vi "Deserialize Core.vi"(8 "error in (no error)":errorcluster, 10 "Serialized Attributes":string, 11 "Serialize in":refnum<class "Update Number Msg.lvclass">) -> (0 "error out":errorcluster, 3 "Serialize out":refnum<class "Update Number Msg.lvclass">)   [LabVIEW 2020, in "Chat Window.lvlib" / "Update Number Msg.lvclass"]
uses:
  Update Number Msg.lvclass
  Update Number Msg.lvclass/Update Number Msg.ctl
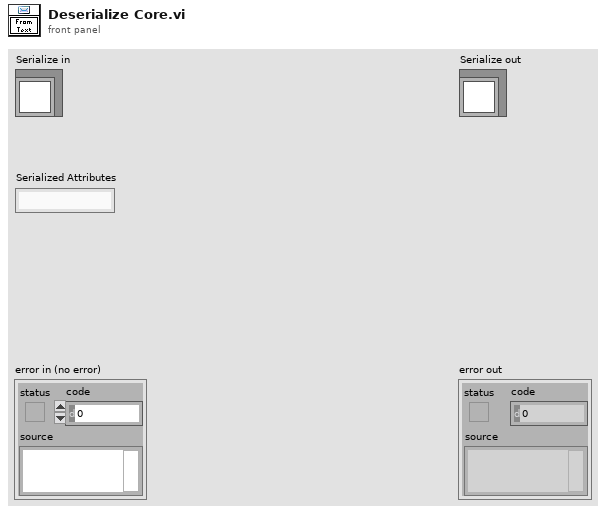
[diagram p1: front panel]
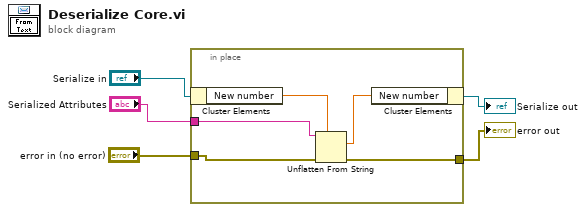
[diagram p0: block diagram]
diagram:
  n1 = in-place "In Place Element Structure" {
    in-place-border: "Serialized Attributes" -> [w9]
    in-place-border: "error in (no error)" -> [w8]
    in-place-border: [w6] -> w2
    n2 = in-place-cluster #1("Serialize in") -> ("New number"=w10:dbl)
    n3 = Unflatten From String(type=w10, binary string=w9, error in (no error)=w8) -> (value=w7:dbl, error out=w6:errorcluster)  [unwired: 2 in, 1 out]
    n4 = in-place-cluster #1("New number"=w7) -> (→"Serialize out":refnum<class "Update Number Msg.lvclass">)
  }
  "error out" <- w2
